vi "Actor Core.vi"(8 "error in":errorcluster, 11 "Simulated Water Level":refnum<class "Simulated Water Level.lvclass">) -> (0 "error out":errorcluster, 3 "Actor out":refnum<class "Actor.lvclass">)   [LabVIEW 2018, in "Simulated Water Level.lvclass"]
doc: "This is Actor Core.vi, the main message handling loop for Actors. An actor usually just sits in this loop and processes messages as they arrive. Any error returned by the message Do.vi call will stop the loop, with error code 43 as the canonical signal to stop with no error sent to caller. Descendants may override that in Handle Error.vi."
uses:
  Simulated Water Level.lvclass
  <vilib>/ActorFramework/Actor/Actor.lvclass
  Cooler Plug-Ins/Simulated Evaporative Cooler.lvclass/Simulation Data_Global.vi
  Water Level/Water Level.lvclass
  Cooler Plug-Ins/Simulated Evaporative Cooler.lvclass/Simulated Evaporative Cooler.lvclass
panel:
  out "stop signal":bool
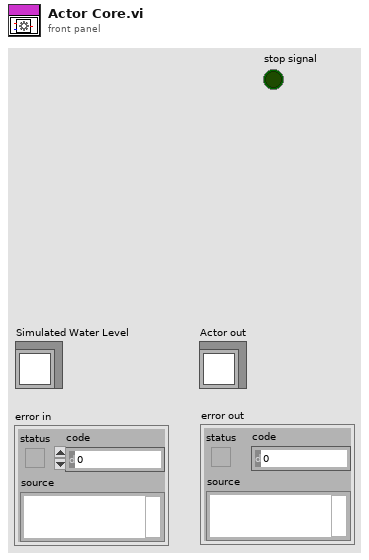
[diagram p1: front panel]
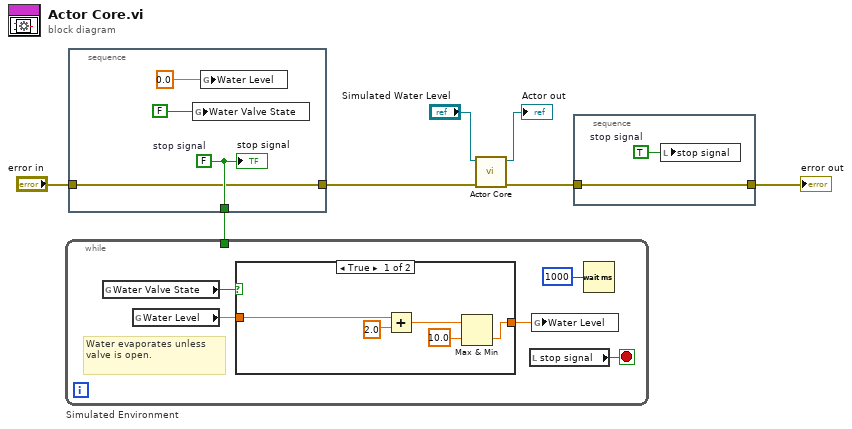
[diagram p0: block diagram]
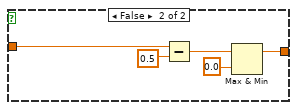
[diagram p2: hidden frame]
diagram:
  n1 = stacked-sequence {
    tunnel: [w11] -> w7
    tunnel: [w10] -> w4
    tunnel: "error in" -> [w10]
    frame #0 {
      w11 = FALSE  # stop signal
      n2 = global write "Simulation Data_Global.vi" "Water Valve State"(FALSE ("Water Valve State")) -> ()
      n3 = global write "Simulation Data_Global.vi" "Water Level"(0.0 ("Water Level")) -> ()
      "stop signal" <- w11
    }
  }
  n4 = while "Simulated Environment" {
    tunnel: w7 -> [_]
    stop <- w16 stop-if-true
    # "Water evaporates unless valve is open."
    n5 = global read "Simulation Data_Global.vi" "Water Valve State"() -> (w14:bool)
    n6 = global read "Simulation Data_Global.vi" "Water Level"() -> (w13:dbl)
    n7 = case shown="True" w14 {
      tunnel: w13 -> [w18 w23]
      tunnel: [w17 w22] -> w12
      frame True {
        n8 = Add(x=w18, y=2.0) -> (x+y=w20:dbl)
        n9 = Max & Min(x=w20, y=10.0) -> (min(x,y)=w17:dbl)  [unwired: 1 out]
      }
      frame False {
        n10 = Subtract(x=w23, y=0.5) -> (x-y=w25:dbl)
        n11 = Max & Min(x=w25, y=0.0) -> (max(x,y)=w22:dbl)  [unwired: 1 out]
      }
    }
    n12 = local read "stop signal"() -> (w16:bool)
    n13 = global write "Simulation Data_Global.vi" "Water Level"(w12) -> ()
    n14 = Wait (ms)(milliseconds to wait=u32 1000) -> ()  [unwired: 1 out]
  }
  n15 = call-parent "Actor Core.vi"("error in"=w4, "Timed Loop Controller"="Simulated Water Level") -> ("error out"=w1:errorcluster, "Actor out"=→"Actor out":refnum<class "Actor.lvclass">)  [unwired: 8 in]
  n16 = stacked-sequence {
    tunnel: [w27] -> w2
    tunnel: w1 -> [w27]
    frame #0 {
      w28 = TRUE  # stop signal
      n17 = local write "stop signal"(w28) -> ()
    }
  }
  "error out" <- w2
